vi "Wait for VeriStand Host.vi"   [LabVIEW 2019, in "LRUTS FPGA IP.lvlib"]
uses:
  LRUTS FPGA IP.lvlib
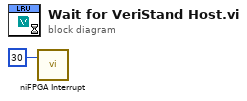
[diagram p0: block diagram]
diagram:
  n1 = call <vilib>:"niFPGA Interrupt.vi"("IRQ Number (0)"=u8 30) -> ()  [unwired: 2 in]
